vi "Get NI-SWITCH Resource.vi"(8 "error in":errorcluster, 11 "ni-switch custom device in":T1 format="%.0x") -> (0 "error out":errorcluster, 2 "resource":string, 3 "ni-switch custom device out":T1 format="%.0x")   [LabVIEW 2017, in "NI-SWITCH Scripting.lvlib"]
doc: "Returns the configured product name for the SLSC Switch custom device."
uses:
  NI-SWITCH Scripting.lvlib
  <vilib>/NI Veristand/Custom Device API/Custom Device Item Ref.ctl
  SLSC Scripting Constants.vi
  <vilib>/NI Veristand/Custom Device API/Get Item Property (String).vi
  <vilib>/NI VeriStand/Custom Device API/Custom Device API.lvlib
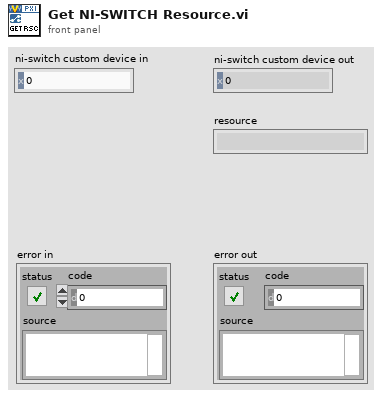
[diagram p1: front panel]
types:
  T1 = typedef "Custom Device API.lvlib/Custom Device Item Ref.ctl" = u64
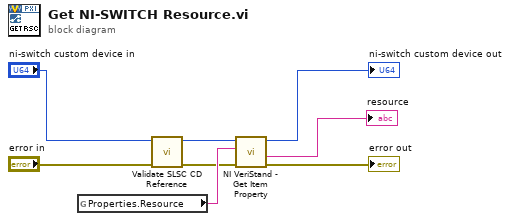
[diagram p0: block diagram]
diagram:
  n1 = global read "SLSC Scripting Constants.vi" "Properties.Resource"() -> (w6:string)
  n2 = call "Validate SLSC CD Reference.vi"("error in"="error in", "ni-switch custom device in"="ni-switch custom device in") -> ("error out"=w3:errorcluster, "ni-switch custom device out"=w1:T1)  [unwired: 8 in]
  n3 = call-poly <vilib>:"NI VeriStand - Get Item Property.vi"("error in (no error)"=w3, "Property Name"=w6, "Item Ref in"=w1) -> ("error out"=→"error out":errorcluster, "Value"=→"resource":string, "Item Ref out"=→"ni-switch custom device out":T1)  [unwired: 5 in, 1 out]
